vi "uTTA_SetMode.vi"(4 "error in":errorcluster, 6 "OperatingMode":T1, 7 "VISA Refnum in":refnum<visa-resource-name>) -> (0 "error out":errorcluster, 2 "Received":string, 3 "VISA Refnum out":refnum<visa-resource-name>)   [LabVIEW 2021]
uses:
  CTL_uTTA_OperatingMode.ctl
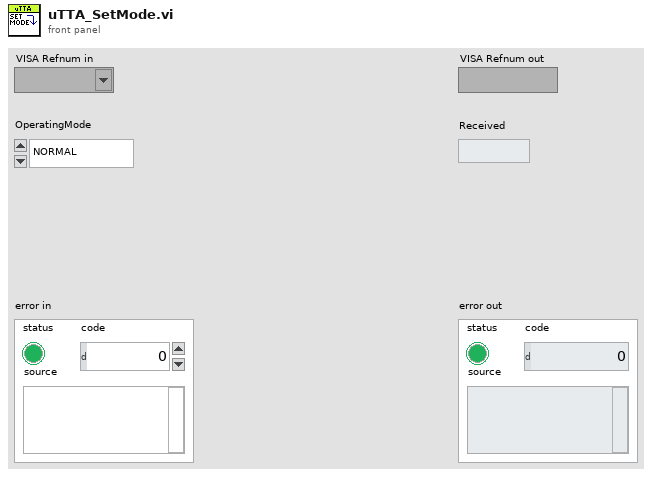
[diagram p1: front panel]
types:
  T1 = typedef "CTL_uTTA_OperatingMode.ctl" = enum16{"NORMAL", "CALIBRATION"}
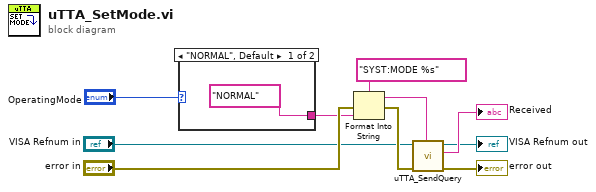
[diagram p0: block diagram]
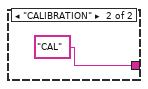
[diagram p2: hidden frame]
diagram:
  n1 = case shown="\"NORMAL\", Default" "OperatingMode" {
    tunnel: ["NORMAL" ("input 1") "CAL" ("input 1")] -> w1
    frame "NORMAL", Default {
    }
    frame "CALIBRATION" {
    }
  }
  n2 = Format Into String(format string="SYST:MODE %s", error in="error in", w1) -> (resulting string=w7:string, error out=w9:errorcluster)  [unwired: 1 in]
  n3 = call "uTTA_SendQuery.vi"("Send String"=w7, "error in (no error)"=w9, "VISA Refnum in"="VISA Refnum in") -> ("error out"=→"error out":errorcluster, "Received"=→"Received":string, "VISA Refnum out"=→"VISA Refnum out":refnum<visa-resource-name>)  [unwired: 6 in]
